vi "read_params.vi"(8 "error in (no error)":errorcluster, 11 "RidgeClassifierCV in":refnum<class "RidgeClassifierCV.lvclass">) -> (0 "error out":errorcluster, 2 "params":T1={"alphas"=[0.1, 1.0, 10.0], "fit_intercept"=TRUE, "normalize"=FALSE, "scoring"="None", "cv"=5.0, "class_weight"={"class_weight_type"="None", "class_weight_dict"="{0:1.2,1:0.8,2:1.0}"}, "store_cv_values"=FALSE}, 3 "RidgeClassifierCV out":refnum<class "RidgeClassifierCV.lvclass">)   [LabVIEW 2020, in "RidgeClassifierCV.lvclass"]
uses:
  RidgeClassifierCV.lvclass
  Controls/ridge_classifier_cv_params.ctl
  RidgeClassifierCV.lvclass/RidgeClassifierCV.ctl
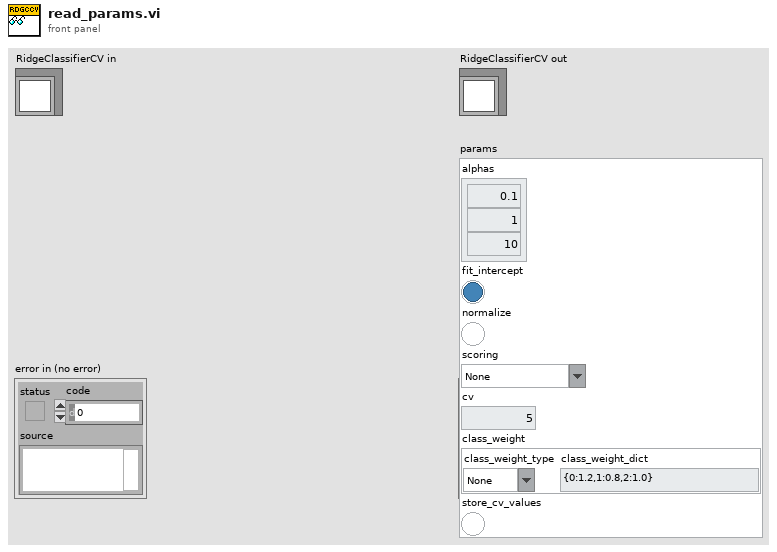
[diagram p1: front panel]
types:
  T1 = typedef "ridge_classifier_cv_params.ctl" = cluster{"alphas":dbl[], "fit_intercept":bool, "normalize":bool, "scoring":string, "cv":dbl, "class_weight":cluster{"class_weight_type":string, "class_weight_dict":string}, "store_cv_values":bool}
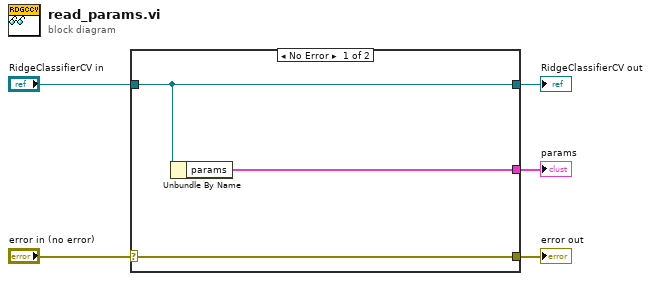
[diagram p0: block diagram]
diagram:
  n1 = case shown="No Error" "error in (no error)" {
    selector: "error in (no error)" -> [w8 w9]
    tunnel: [w8 w9] -> w4
    tunnel: [w7 w10] -> w2
    tunnel: "RidgeClassifierCV in" -> [w7 w10]
    tunnel: [w6 _] -> w1
    frame No Error {
      n2 = Unbundle By Name(w7) -> ("params"=w6:T1)
    }
    frame Error {
    }
  }
  "error out" <- w4
  "RidgeClassifierCV out" <- w2
  "params" <- w1
